vi "IsVI.vi"(0 "ProjectItem Refnum":refnum<vi>) -> (2 "IsVI?":bool)   [LabVIEW 2014, in "_ProjectItemsUtilities.lvlib"]
uses:
  _ProjectItemsUtilities.lvlib
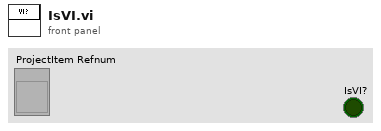
[diagram p1: front panel]
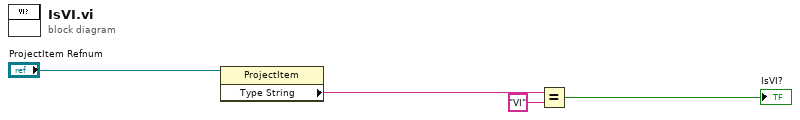
[diagram p0: block diagram]
diagram:
  n1 = property class="ProjectItem"(reference="ProjectItem Refnum") -> ("Type String"=w2:string)  [unwired: 1 in, 2 out]
  n2 = Equal?(x=w2, y="VI") -> (x = y?=→"IsVI?":bool)
